vi "Write Digital Port.vi"(8 "error in (no error)":errorcluster, 10 "DOs":bool[](array[boolean]), 11 "Digital Output in":refnum<class "DO.lvclass">) -> (0 "error out":errorcluster, 3 "Digital Output out":refnum<class "DO.lvclass">)   [LabVIEW 2025, in "Interface.lvlib" / "DO.lvclass"]
uses:
  DO.lvclass
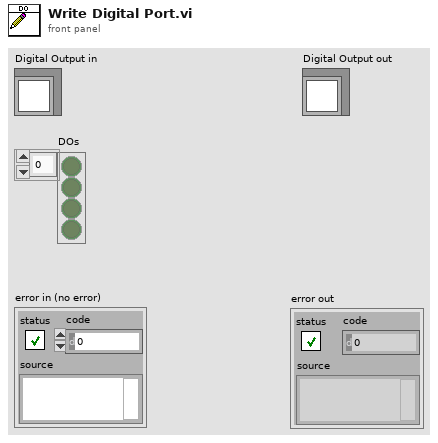
[diagram p1: front panel]
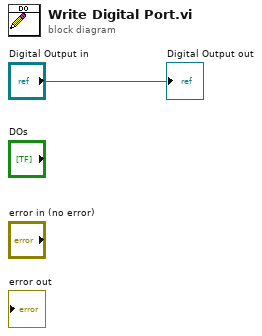
[diagram p0: block diagram]
diagram:
  "Digital Output out" <- "Digital Output in"
